vi "Server_Queue Release.vi"(8 "error in":errorcluster, 11 "Main Queue":T1) -> (0 "error out":errorcluster)   [LabVIEW 2018, in "Cloud Server.lvlib"]
uses:
  Cloud Server.lvlib
  Data Def/Server_Main Queue.ctl
  Data Def/Server_Server Write Queue Data.ctl
  Data Def/Server_Main Loop Queue Data.ctl
  Data Def/Server_Main Loop State.ctl
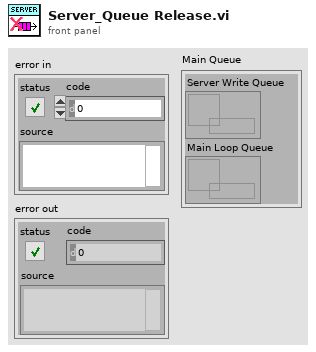
[diagram p1: front panel]
types:
  T1 = typedef "Cloud Server.lvlib/Server_Main Queue.ctl" = cluster{"Server Write Queue":refnum<queue>, "Main Loop Queue":refnum<queue>}
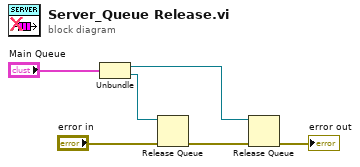
[diagram p0: block diagram]
diagram:
  n1 = Unbundle("Main Queue") -> ("Server Write Queue"=w3:refnum<queue>, "Main Loop Queue"=w5:refnum<queue>)
  n2 = Release Queue(queue=w5, error in (no error)="error in") -> (error out=w4:errorcluster)  [unwired: 1 in, 2 out]
  n3 = Release Queue(queue=w3, error in (no error)=w4) -> (error out=→"error out":errorcluster)  [unwired: 1 in, 2 out]
